vi "is_dbl.vi"(11 "data in":string) -> (1 "confirmed?":bool, 3 "data out":variant)   [LabVIEW 2020, in "configuration-data.lvclass"]
uses:
  configuration-data.lvclass
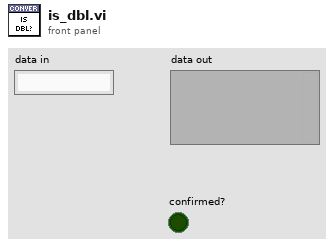
[diagram p1: front panel]
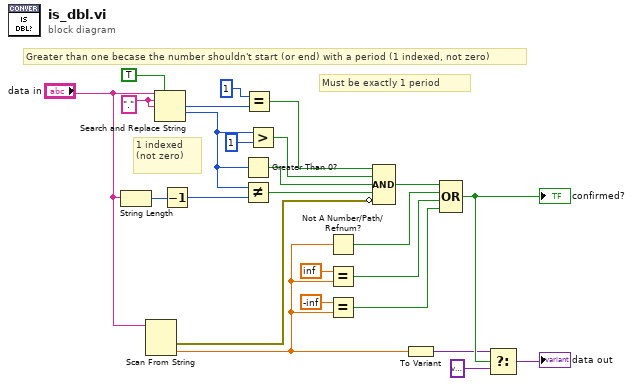
[diagram p0: block diagram]
diagram:
  w22 = "." ("search string/char (-)")
  # "Must be exactly 1 period"
  # "1 indexed (not zero)"
  # "Greater than one becase the number shouldn't start (or end) with a period (1 indexed, not zero)"
  n1 = String Length(string="data in") -> (length=w25:i32)
  n2 = Scan From String(input string="data in") -> (error out=w17:errorcluster, output 1=w5:dbl)  [unwired: 4 in, 2 out]
  n3 = Search and Replace String(replace all?=TRUE ("replace all? (F)"), input string="data in", search string=w22, replace string=w22) -> (number of replacements=w20:i32, offset past replacement=w15:i32)  [unwired: 4 in, 2 out]
  n4 = Decrement(x=w25) -> (x-1=w24:i32)
  n5 = Greater Than 0?(x=w15) -> (x > 0?=w16:bool)
  n6 = Not Equal?(x=w15, y=w24) -> (x != y?=w18:bool)
  n7 = Equal?(x=1, y=w20) -> (x = y?=w12:bool)
  n8 = Greater?(x=w15, y=1 ("x")) -> (0:w13:bool)
  n9 = Not A Number/Path/Refnum?(number/path/refnum=w5) -> (NaN/Path/Refnum?=w8:bool)
  n10 = Equal?(x=inf, y=w5) -> (x = y?=w7:bool)
  n11 = Equal?(x=-inf, y=w5) -> (x = y?=w6:bool)
  n12 = Compound Arithmetic op=AND(w12, w13, w16, w18, invert w17) -> (w9:bool)
  n13 = To Variant(anything=w5) -> (Variant=w3:variant)
  n14 = Compound Arithmetic op=OR(w9, w8, w7, w6) -> (w4:bool)
  "confirmed?" <- w4
  n15 = Select(t=w3, s=w4, f=variant) -> (s? t:f=→"data out":variant)
